vi "Read 2D Strings From Config.vi"(11 "key":string="TextIcons.Abbreviate") -> (3 "2D array strings":string[][](array[string]))   [LabVIEW 2020, in "Text-Based VI Icon.lvlib"]
uses:
  Text-Based VI Icon.lvlib
  <resource>/dialog/lvconfig.llb/LV Config Read String.vi
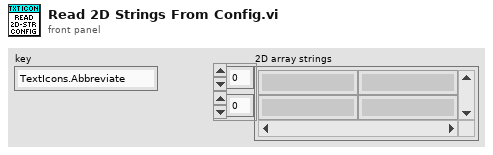
[diagram p1: front panel]
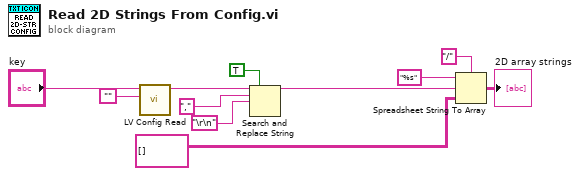
[diagram p0: block diagram]
diagram:
  n1 = call-poly <resource>:"LV Config Read.vi"("default value"="", "key"="key") -> ("value"=w5:string)  [unwired: 3 in, 2 out]
  n2 = Search and Replace String(replace all?=TRUE ("replace all? (F)"), input string=w5, search string=",", replace string="\r\n") -> (result string=w1:string)  [unwired: 4 in, 3 out]
  n3 = Spreadsheet String To Array(delimiter (Tab)="/", format string="%s", spreadsheet string=w1, array type (2D Dbl)=string[][] []) -> (array=→"2D array strings":string[][])
